vi "C_A_text.vi"() -> (0 "array":dbl[](array[numeric]))   [LabVIEW 2020]
panel:
  out "size(s) 2":i32
  in  "Путь к записи сигнала":path=path "C:/Users/ira_1/OneDrive/Рабочий стол/GPS-TX-RX/code.txt"
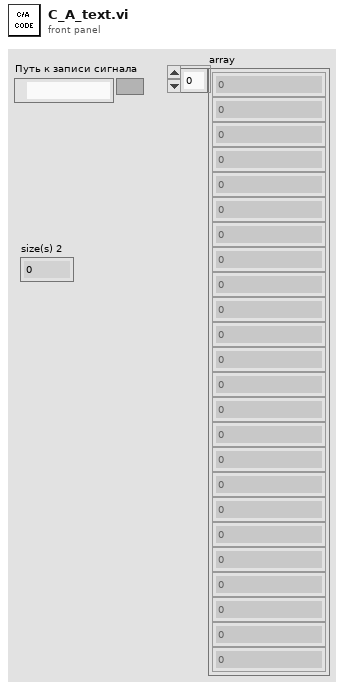
[diagram p1: front panel]
types:
  T1 = enum16{"open", "replace", "create", "open or create", "replace or create", "replace or create with confirmation"}
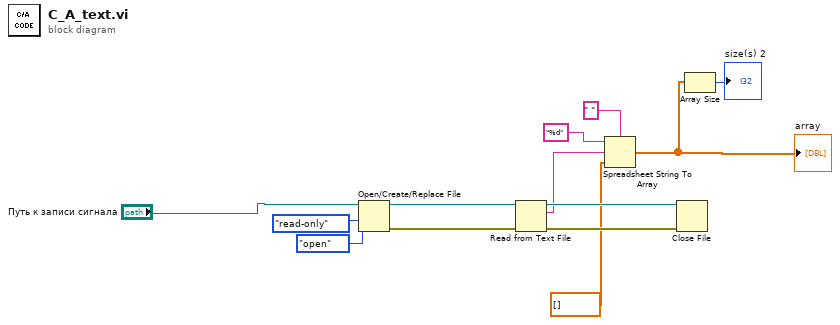
[diagram p0: block diagram]
diagram:
  n1 = Open/Create/Replace File(file path (use dialog)="Путь к записи сигнала", operation (0:open)=T1."open", access (0:read/write)=enum16{"read/write", "read-only", "write-only"}."read-only") -> (refnum out=w13:refnum<file>, error out=w12:errorcluster)  [unwired: 3 in, 1 out]
  n2 = Read from Text File(file (use dialog)=w13, error in=w12) -> (refnum out=w9:refnum<file>, text=w5:string, error out=w8:errorcluster)  [unwired: 2 in, 1 out]
  n3 = Spreadsheet String To Array(delimiter (Tab)=" ", format string="%d", spreadsheet string=w5, array type (2D Dbl)=dbl[] []) -> (array=w2:dbl[])
  "array" <- w2
  n4 = Close File(refnum=w9, error in=w8) -> ()  [unwired: 2 out]
  n5 = Array Size(array=w2) -> (size(s)=→"size(s) 2":i32)
